vi "setInstName.vi"(8 "error in (no error)":errorcluster, 11 "OptCtrl in":refnum<class "OptCtrl.lvclass">) -> (0 "error out":errorcluster, 3 "OptCtrl out":refnum<class "OptCtrl.lvclass">)   [LabVIEW 2016, in "OptCtrl.lvclass"]
doc: "Set the instrument name (e.g. lsst or comcam)."
uses:
  OptCtrl.lvclass
  OptCtrl.lvclass/OptCtrl.ctl
panel:
  in  "Inst Name":string="lsst"
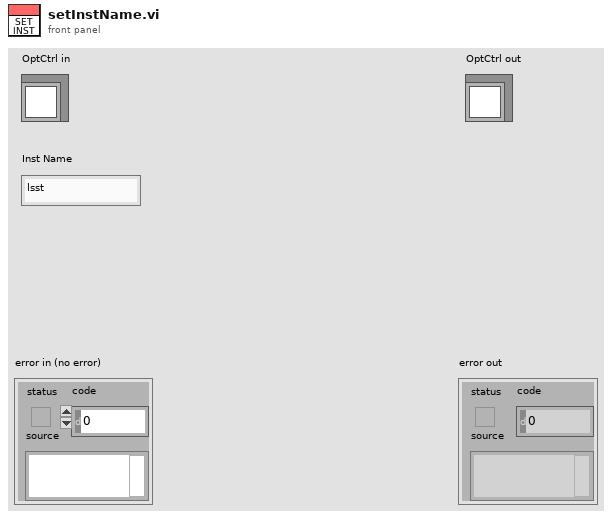
[diagram p1: front panel]
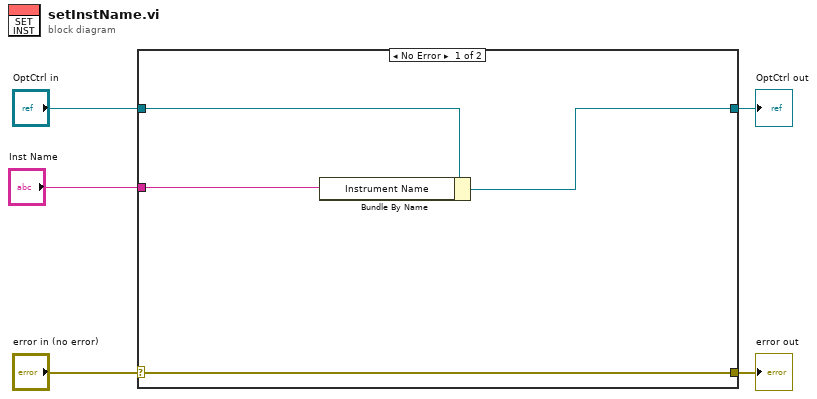
[diagram p0: block diagram]
diagram:
  n1 = case shown="No Error" "error in (no error)" {
    selector: "error in (no error)" -> [w9 w11]
    tunnel: [w9 w11] -> w4
    tunnel: [w6 w10] -> w2
    tunnel: "OptCtrl in" -> [w7 w10]
    tunnel: "Inst Name" -> [w8 _]
    frame No Error {
      n2 = Bundle By Name(cluster=w7, "Instrument Name"=w8) -> (w6:refnum<class "OptCtrl.lvclass">)
    }
    frame Error {
    }
  }
  "error out" <- w4
  "OptCtrl out" <- w2
